vi "OEE_SCREEN_2_recolor_OEE.vi"(1 "OEE_actual_field_reference":refnum<vi>, 2 "OEE_actual_value":string) -> ()   [LabVIEW 2019]
uses:
  FGV/SQL_raw_data/FGV_OEE_SQL_raw_data.ctl
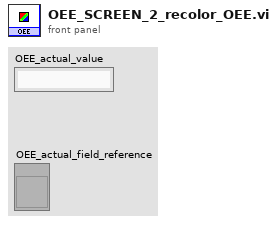
[diagram p1: front panel]
types:
  T1 = typedef "FGV_OEE_SQL_raw_data.ctl" = enum16{"initialize", "set_reference_name", "set_timestamp", "set_OK_NOK_count", "set_config_info", "set_cycle_time_and_pace", "set_last_operator", "set_availability", "set_hourly_ok_count", "set_targets", "get_all_info"}
  T2 = typedef "OEE_SQL_raw_data.ctl" = cluster{"reference_name":string, "data_timestamp":timestamp, "OK_NOK_count":string[][], "config_info":string[], "pace":string[][], "last_operator":string[][], "availability":string[], "hourly_ok_count":string[][], "shift_start":i8, "shift_end":i8, "TAKT":u16, "FTTH_target":u16, "OEE_target":u16, "BOTTLENECK_station":u16, "targets_hourly":u16[], "target_shift":u16}
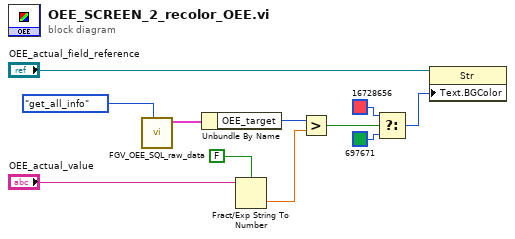
[diagram p0: block diagram]
diagram:
  n1 = call "FGV_OEE_SQL_raw_data.vi"("options"=FGV_OEE_SQL_raw_data."get_all_info") -> ("SQL_raw_data_out"=w2:T2)  [unwired: 9 in, 1 out]
  n2 = Unbundle By Name(w2) -> ("OEE_target"=w5:u16)
  n3 = Fract/Exp String To Number(use system decimal point (T)=FALSE, string="OEE_actual_value") -> (number=w6:dbl)  [unwired: 2 in, 1 out]
  n4 = Greater?(x=w5, y=w6) -> (0:w9:bool)
  n5 = Select(t=u32 16728656, s=w9, f=u32 697671) -> (s? t:f=w11:u32)
  n6 = property class="Str"(reference="OEE_actual_field_reference", "Text.BGColor"=w11) -> ()  [unwired: 1 in, 2 out]
